vi "PointsEqual.vi"(10 "Point2D_2":T1={"X"=-17.320509, "Y"=-40.0, "Slope"=32.41122055053711}, 11 "Point2D_1":T1={"X"=1.2289006, "Y"=-0.30202582, "Slope"=74.3662109375}) -> (3 "Equal?":bool)   [LabVIEW 2014]
uses:
  TypeDefs/Point2DwSlope.ctl
panel:
  in  "Tolerance":sgl=1e-06
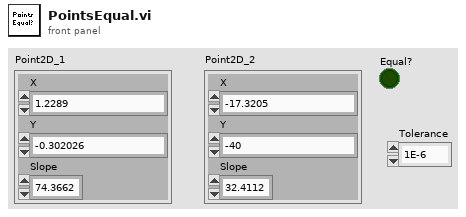
[diagram p1: front panel]
types:
  T1 = typedef "Point2DwSlope.ctl" = cluster{"X":sgl, "Y":sgl, "Slope":dbl}
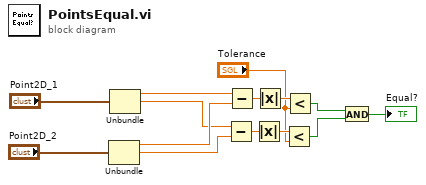
[diagram p0: block diagram]
diagram:
  n1 = Unbundle("Point2D_2") -> ("X"=w10:sgl, "Y"=w4:sgl)  [unwired: 1 out]
  n2 = Unbundle("Point2D_1") -> ("X"=w11:sgl, "Y"=w5:sgl)  [unwired: 1 out]
  n3 = Subtract(x=w5, y=w4) -> (x-y=w6:sgl)
  n4 = Subtract(x=w11, y=w10) -> (x-y=w9:sgl)
  n5 = Absolute Value(x=w6) -> (abs(x)=w7:sgl)
  n6 = Absolute Value(x=w9) -> (abs(x)=w8:sgl)
  n7 = Less?(x=w7, y="Tolerance") -> (x < y?=w1:bool)
  n8 = Less?(x=w8, y="Tolerance") -> (x < y?=w2:bool)
  n9 = And(x=w2, y=w1) -> (x .and. y?=→"Equal?":bool)
